vi "Configure Offset and Limits (Adjacent Channel Power).vi"(0 "VISA resource name":refnum<visa-resource-name>, 1 "Enable Auto Reference Bandwidth List":bool[](array[boolean])=[FALSE, FALSE, FALSE, FALSE, FALSE, FALSE], 5 "Reference Bandwidth List":dbl[](array[numeric])=[2000000.0, 2000000.0, 2000000.0, 2000000.0, 2000000.0, 2000000.0], 7 "Enable Offset Frequency List":bool[](array[boolean])=[FALSE, FALSE, FALSE, FALSE, FALSE, FALSE], 9 "Offset Frequency List":dbl[](array[numeric])=[3000000.0, 3000000.0, 3000000.0, 3000000.0, 3000000.0, 3000000.0], 11 "error in (no error)":errorcluster, 12 "Enable Auto Offset Frequency List":bool[](array[boolean])=[FALSE, FALSE, FALSE, FALSE, FALSE, FALSE]) -> (4 "VISA resource name out":refnum<visa-resource-name>, 15 "error out":errorcluster)   [LabVIEW 2022 SP3, in "Agilent N934X Series.lvlib"]
doc: "Configures the offset frequency under the offsets and limits for Adjacent Channel Power measurement type.\n\nNote:\nThis VI is only applicable for N9321C, N9322C, N9323C, N9324C models"
uses:
  <instrlib>/Agilent N934X Series/Agilent N934X Series.lvlib
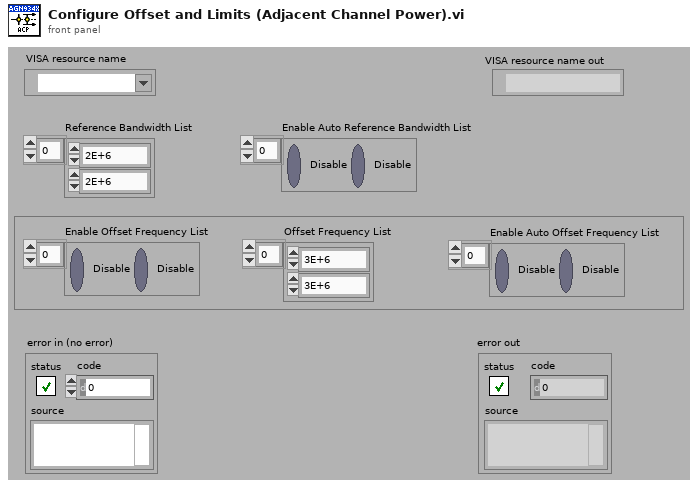
[diagram p1: front panel]
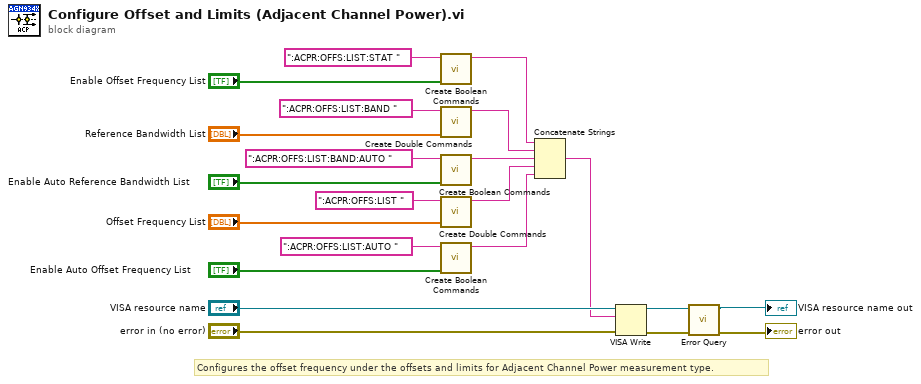
[diagram p0: block diagram]
diagram:
  # "Configures the offset frequency under the offsets and limits for Adjacent Channel Power measurement type."
  n1 = call <instrlib>:"Create Boolean Commands.vi"("Boolean States"="Enable Offset Frequency List", "Command"=":ACPR:OFFS:LIST:STAT " ("format string")) -> ("Result String"=w1:string)  [unwired: 9 in]
  n2 = call <instrlib>:"Create Double Commands.vi"("Double Values"="Reference Bandwidth List", "Commands"=":ACPR:OFFS:LIST:BAND " ("format string")) -> ("Result"=w15:string)  [unwired: 9 in]
  n3 = call <instrlib>:"Create Boolean Commands.vi"("Boolean States"="Enable Auto Reference Bandwidth List", "Command"=":ACPR:OFFS:LIST:BAND:AUTO " ("format string")) -> ("Result String"=w3:string)  [unwired: 9 in]
  n4 = call <instrlib>:"Create Double Commands.vi"("Double Values"="Offset Frequency List", "Commands"=":ACPR:OFFS:LIST " ("format string")) -> ("Result"=w4:string)  [unwired: 9 in]
  n5 = call <instrlib>:"Create Boolean Commands.vi"("Boolean States"="Enable Auto Offset Frequency List", "Command"=":ACPR:OFFS:LIST:AUTO " ("format string")) -> ("Result String"=w5:string)  [unwired: 9 in]
  n6 = Concatenate Strings(w1, w15, w3, w4, w5) -> (w20:string)
  n7 = VISA Write(VISA resource name="VISA resource name", write buffer=w20, error in (no error)="error in (no error)") -> (VISA resource name out=w18:refnum<visa-resource-name>, error out=w19:errorcluster)  [unwired: 1 out]
  n8 = call <instrlib>:"Error Query.vi"("error in (no error)"=w19, "VISA resource name"=w18) -> ("error out"=→"error out":errorcluster, "VISA resource name out"=→"VISA resource name out":refnum<visa-resource-name>)  [unwired: 6 in, 2 out]
